vi "LabviewAMADTest.vi"() -> ()   [LabVIEW 2017]
uses:
  ADAM-4050DLL.dll
panel:
  in  "值_7":bool
  in  "DO7":bool
  in  "值_6":bool
  in  "DO6":bool
  in  "值_5":bool
  in  "DO5":bool
  in  "值_4":bool
  in  "DO4":bool
  in  "值_3":bool
  in  "DO3":bool
  in  "值_2":bool
  in  "DO2":bool
  in  "?":bool
  in  "DO1":bool
  out "inputresut":string[](array[string])
  in  "input":bool[](array[boolean])=[FALSE, FALSE, FALSE, FALSE, FALSE, FALSE, FALSE, FALSE]
  in  "?":bool
  in  "DO0":bool
  in  "停止 2":bool
  out "str_DO":string[](array[string])
  out "str_DI":string[](array[string])
  in  "停止":bool
  out "m_iDOTotalX":i32
  out "m_iDITotalX":i32
  # "值_0"
  # "值_1"
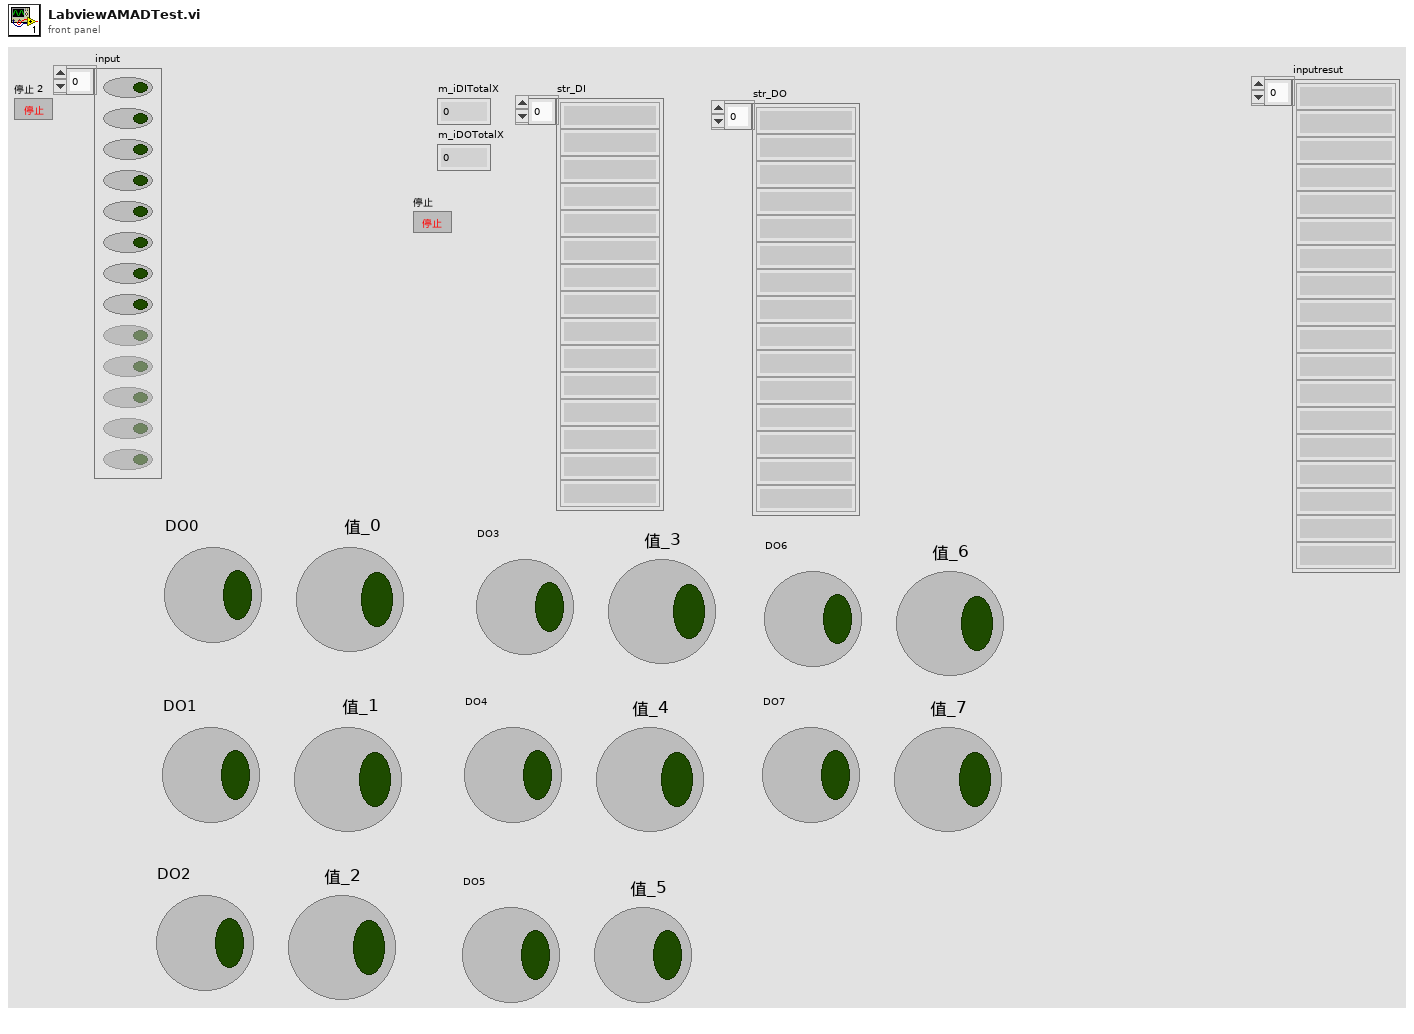
[diagram p1: front panel]
types:
  T1 = typedef "Semaphore RefNum" = refnum<k1>
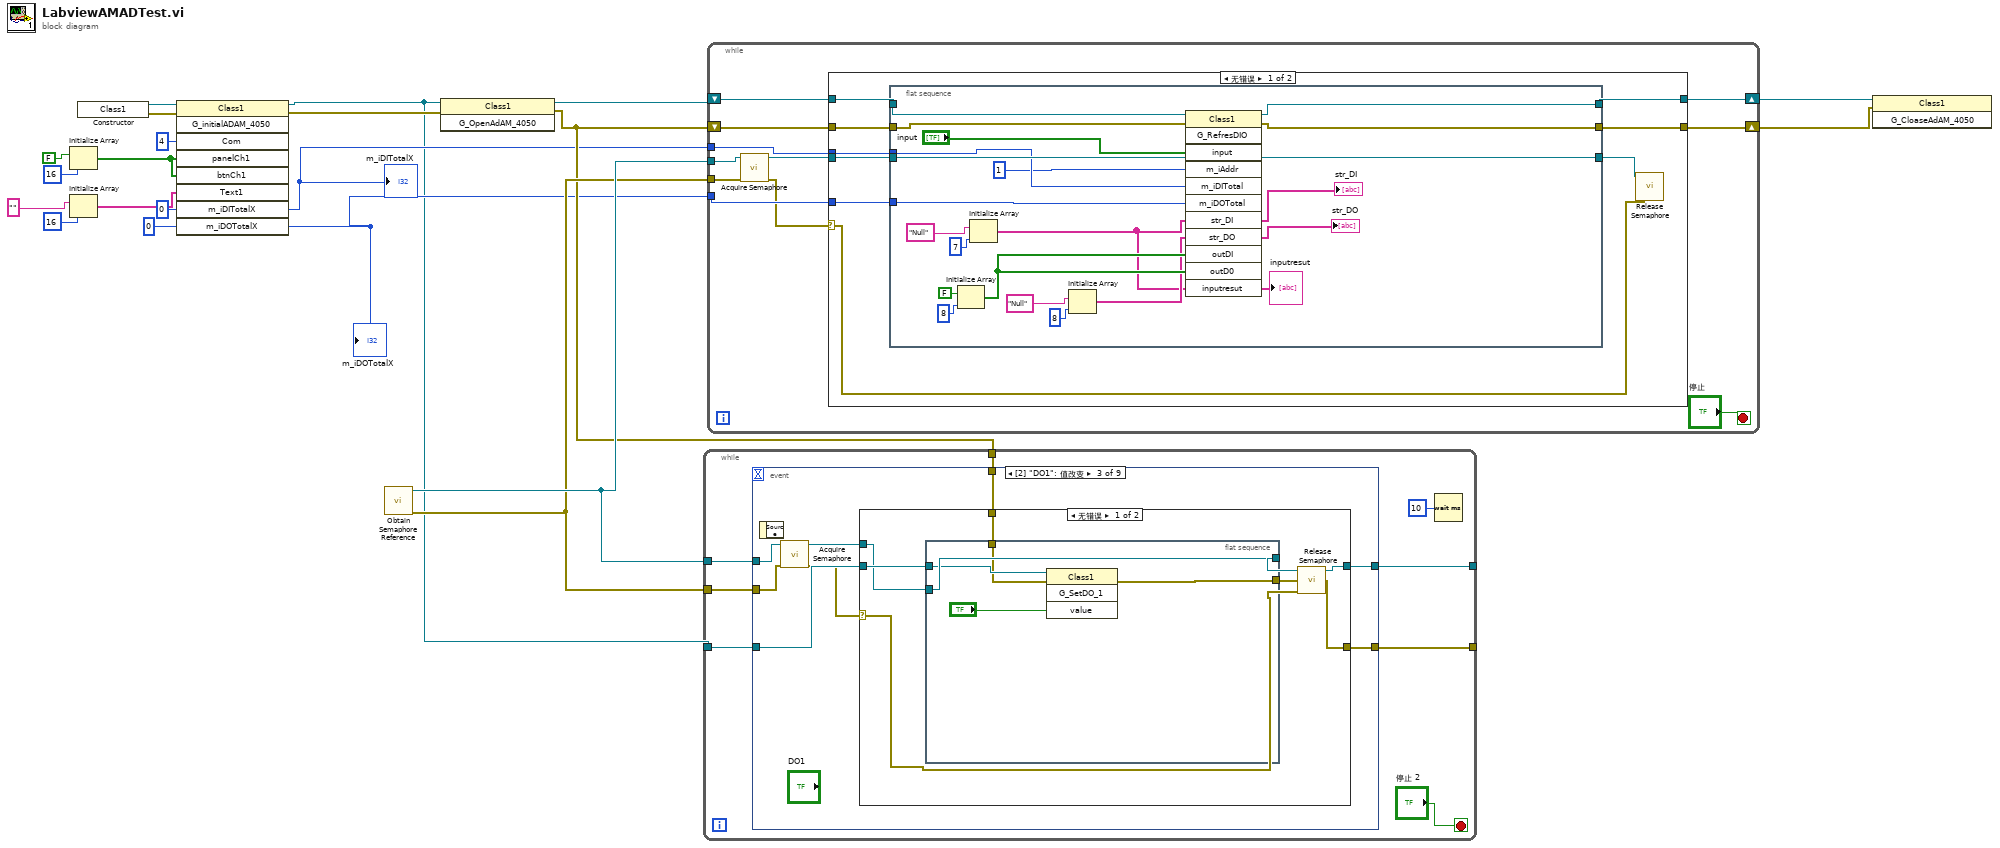
[diagram p0: block diagram]
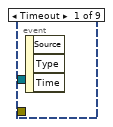
[diagram p2: hidden frame]
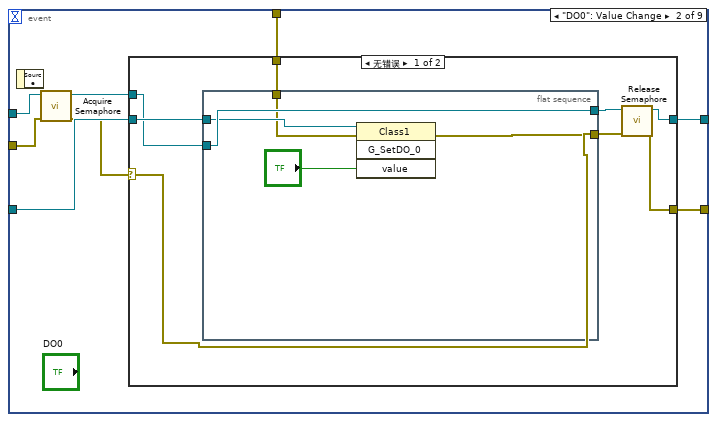
[diagram p3: hidden frame]
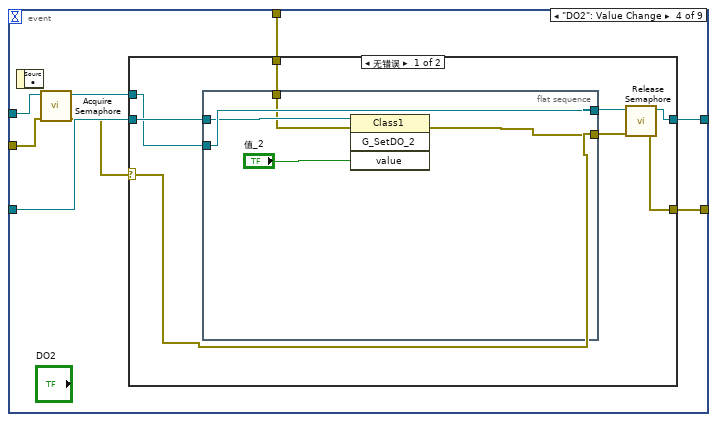
[diagram p6: hidden frame]
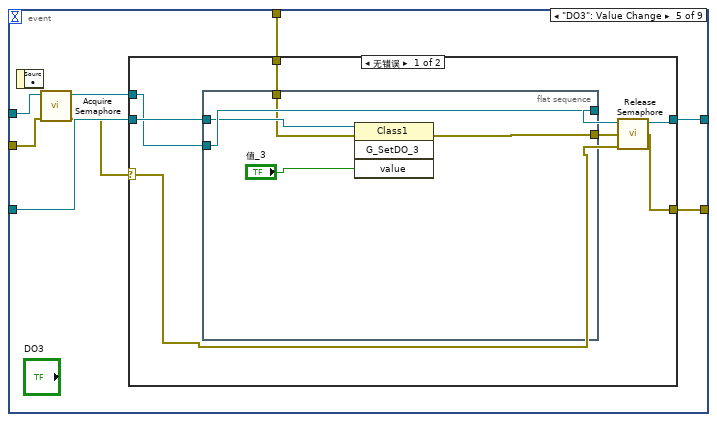
[diagram p8: hidden frame]
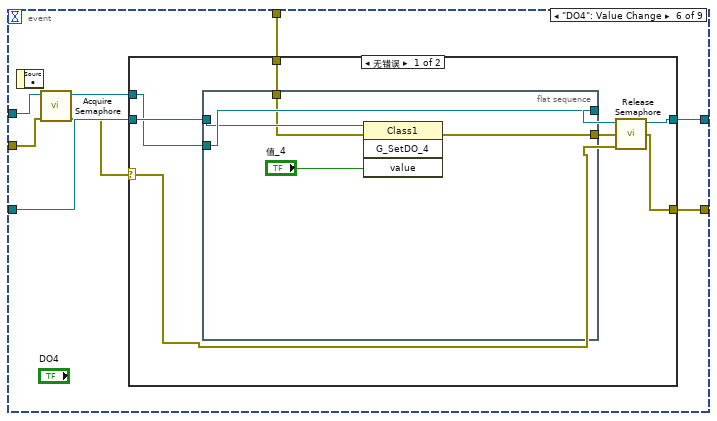
[diagram p10: hidden frame]
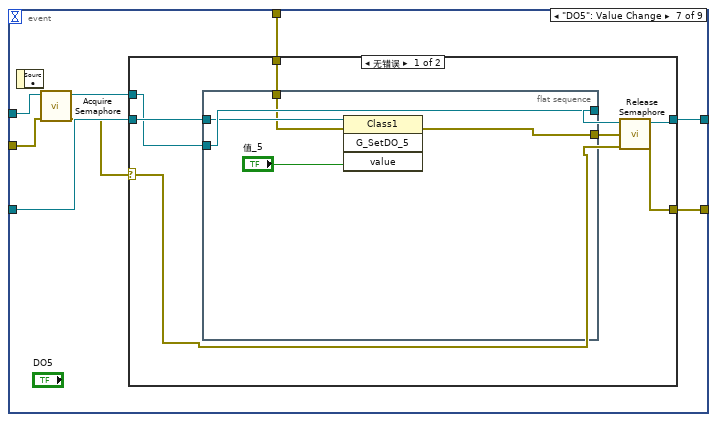
[diagram p12: hidden frame]
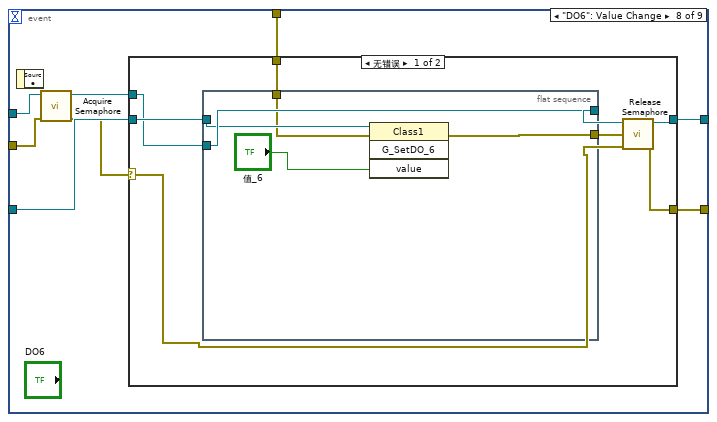
[diagram p14: hidden frame]
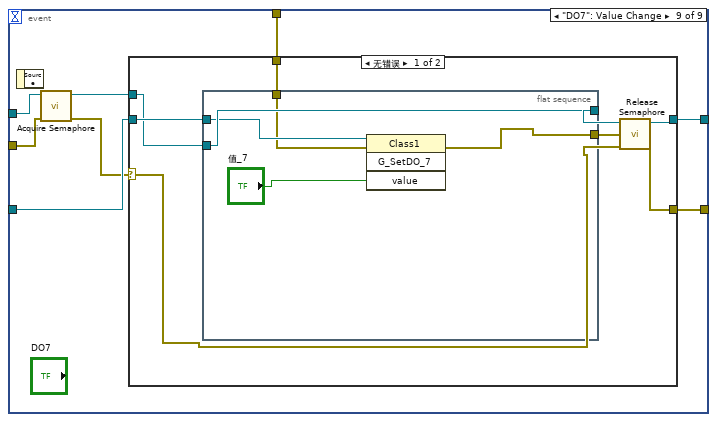
[diagram p16: hidden frame]
diagram:
  n1 = Initialize Array(FALSE, 16 ("维数大小")) -> (w16:bool[])
  n2 = Initialize Array("", 16 ("维数大小")) -> (w13:string[])
  n3 = constructor class="Class1"() -> (reference out=w21:refnum<k24>, error out=w20:errorcluster)  [unwired: 3 in, 1 out]
  n4 = invoke on="调用节点" class="Class1" method="G_initialADAM_4050"(reference=w21, error in=w20, "Com"=4, "panelCh1"=w16, "btnCh1"=w16, "Text1"=w13, "m_iDITotalX"=0, "m_iDOTotalX"=0) -> (reference out=w1:refnum<k24>, error out=w10:errorcluster, "m_iDITotalX"=w5:i32, "m_iDOTotalX"=w4:i32)  [unwired: 1 in, 5 out]
  "m_iDITotalX" <- w5
  "m_iDOTotalX" <- w4
  n5 = call <vilib>:"Obtain Semaphore Reference.vi"() -> ("error out"=w8:errorcluster, "semaphore"=w9:T1)  [unwired: 5 in, 1 out]
  n6 = invoke on="调用节点" class="Class1" method="G_OpenAdAM_4050"(reference=w1, error in=w10) -> (reference out=w7:refnum<k24>, error out=w6:errorcluster)  [unwired: 1 in, 1 out]
  n7 = while {
    tunnel: w9 -> [w27]
    tunnel: w8 -> [w26]
    tunnel: w1 -> [w25]
    tunnel: w6 -> [w24]
    tunnel: [w23] -> _
    tunnel: [w22] -> _
    stop <- "停止 2" stop-if-true
    n8 = event shown="[2] \"DO1\": 值改变" {
      selector: _ -> [_ _ _ _ _ _ _ _ _]
      dyn-events: _ -> [_ _ _ _ _ _ _ _ _]
      timeout: _ -> [_ _ _ _ _ _ _ _ _]
      tunnel: w27 -> [_ w36 w58 w80 w102 w124 w146 w168 w190]
      tunnel: w26 -> [_ w35 w57 w79 w101 w123 w145 w167 w189]
      tunnel: w25 -> [_ w37 w59 w81 w103 w125 w147 w169 w191]
      tunnel: w24 -> [_ w32 w54 w76 w98 w120 w142 w164 w186]
      tunnel: [_ w31 w53 w75 w97 w119 w141 w163 w185] -> w23
      tunnel: [_ w30 w52 w74 w96 w118 w140 w162 w184] -> w22
      event Timeout {
        n9 = event-data() -> ()  [unwired: 1 in, 3 out]
      }
      event "DO0": Value Change {
        n10 = event-data() -> ()  [unwired: 1 in, 1 out]
        n11 = call <vilib>:"Acquire Semaphore.vi"("error in (no error)"=w35, "semaphore"=w36) -> ("error out"=w33:errorcluster, "semaphore out"=w34:T1)  [unwired: 3 in, 1 out]
        n12 = case shown="无错误" w33 {
          selector: w33 -> [w43 w51]
          tunnel: w37 -> [w44 _]
          tunnel: w34 -> [w41 w50]
          tunnel: w32 -> [w40 _]
          tunnel: [w38 w50] -> w31
          tunnel: [w39 w51] -> w30
          frame No Error {
            n13 = flat-sequence {
              tunnel: w44 -> [w48]
              tunnel: w41 -> [w49]
              tunnel: [w49] -> w42
              tunnel: w40 -> [w47]
              tunnel: [w46] -> w39
              frame #0 {
                n14 = invoke class="Class1" method="G_SetDO_0"(reference=w48, error in=w47, "value"="?") -> (error out=w46:errorcluster)  [unwired: 1 in, 3 out]
              }
            }
            n15 = call <vilib>:"Release Semaphore.vi"("error in (no error)"=w43, "semaphore"=w42) -> ("semaphore out"=w38:T1)  [unwired: 4 in, 1 out]
          }
          frame Error {
          }
        }
      }
      event "DO1": Value Change {
        n16 = event-data() -> ()  [unwired: 1 in, 1 out]
        n17 = call <vilib>:"Acquire Semaphore.vi"("error in (no error)"=w57, "semaphore"=w58) -> ("error out"=w55:errorcluster, "semaphore out"=w56:T1)  [unwired: 3 in, 1 out]
        n18 = case shown="无错误" w55 {
          selector: w55 -> [w65 w73]
          tunnel: w59 -> [w66 _]
          tunnel: w56 -> [w63 w72]
          tunnel: w54 -> [w62 _]
          tunnel: [w60 w72] -> w53
          tunnel: [w61 w73] -> w52
          frame No Error {
            n19 = flat-sequence {
              tunnel: w66 -> [w70]
              tunnel: w63 -> [w71]
              tunnel: [w71] -> w64
              tunnel: w62 -> [w69]
              tunnel: [w68] -> w61
              frame #0 {
                n20 = invoke class="Class1" method="G_SetDO_1"(reference=w70, error in=w69, "value"="?") -> (error out=w68:errorcluster)  [unwired: 1 in, 3 out]
              }
            }
            n21 = call <vilib>:"Release Semaphore.vi"("error in (no error)"=w65, "semaphore"=w64) -> ("semaphore out"=w60:T1)  [unwired: 4 in, 1 out]
          }
          frame Error {
          }
        }
      }
      event "DO2": Value Change {
        n22 = event-data() -> ()  [unwired: 1 in, 1 out]
        n23 = call <vilib>:"Acquire Semaphore.vi"("error in (no error)"=w79, "semaphore"=w80) -> ("error out"=w77:errorcluster, "semaphore out"=w78:T1)  [unwired: 3 in, 1 out]
        n24 = case shown="无错误" w77 {
          selector: w77 -> [w87 w95]
          tunnel: w81 -> [w88 _]
          tunnel: w78 -> [w85 w94]
          tunnel: w76 -> [w84 _]
          tunnel: [w82 w94] -> w75
          tunnel: [w83 w95] -> w74
          frame No Error {
            n25 = flat-sequence {
              tunnel: w88 -> [w92]
              tunnel: w85 -> [w93]
              tunnel: [w93] -> w86
              tunnel: w84 -> [w91]
              tunnel: [w90] -> w83
              frame #0 {
                n26 = invoke class="Class1" method="G_SetDO_2"(reference=w92, error in=w91, "value"="值_2") -> (error out=w90:errorcluster)  [unwired: 1 in, 3 out]
              }
            }
            n27 = call <vilib>:"Release Semaphore.vi"("error in (no error)"=w87, "semaphore"=w86) -> ("semaphore out"=w82:T1)  [unwired: 4 in, 1 out]
          }
          frame Error {
          }
        }
      }
      event "DO3": Value Change {
        n28 = event-data() -> ()  [unwired: 1 in, 1 out]
        n29 = call <vilib>:"Acquire Semaphore.vi"("error in (no error)"=w101, "semaphore"=w102) -> ("error out"=w99:errorcluster, "semaphore out"=w100:T1)  [unwired: 3 in, 1 out]
        n30 = case shown="无错误" w99 {
          selector: w99 -> [w109 w117]
          tunnel: w103 -> [w110 _]
          tunnel: w100 -> [w107 w116]
          tunnel: w98 -> [w106 _]
          tunnel: [w104 w116] -> w97
          tunnel: [w105 w117] -> w96
          frame No Error {
            n31 = flat-sequence {
              tunnel: w110 -> [w114]
              tunnel: w107 -> [w115]
              tunnel: [w115] -> w108
              tunnel: w106 -> [w113]
              tunnel: [w112] -> w105
              frame #0 {
                n32 = invoke class="Class1" method="G_SetDO_3"(reference=w114, error in=w113, "value"="值_3") -> (error out=w112:errorcluster)  [unwired: 1 in, 3 out]
              }
            }
            n33 = call <vilib>:"Release Semaphore.vi"("error in (no error)"=w109, "semaphore"=w108) -> ("semaphore out"=w104:T1)  [unwired: 4 in, 1 out]
          }
          frame Error {
          }
        }
      }
      event "DO4": Value Change {
        n34 = event-data() -> ()  [unwired: 1 in, 1 out]
        n35 = call <vilib>:"Acquire Semaphore.vi"("error in (no error)"=w123, "semaphore"=w124) -> ("error out"=w121:errorcluster, "semaphore out"=w122:T1)  [unwired: 3 in, 1 out]
        n36 = case shown="无错误" w121 {
          selector: w121 -> [w131 w139]
          tunnel: w125 -> [w132 _]
          tunnel: w122 -> [w129 w138]
          tunnel: w120 -> [w128 _]
          tunnel: [w126 w138] -> w119
          tunnel: [w127 w139] -> w118
          frame No Error {
            n37 = flat-sequence {
              tunnel: w132 -> [w136]
              tunnel: w129 -> [w137]
              tunnel: [w137] -> w130
              tunnel: w128 -> [w135]
              tunnel: [w134] -> w127
              frame #0 {
                n38 = invoke class="Class1" method="G_SetDO_4"(reference=w136, error in=w135, "value"="值_4") -> (error out=w134:errorcluster)  [unwired: 1 in, 3 out]
              }
            }
            n39 = call <vilib>:"Release Semaphore.vi"("error in (no error)"=w131, "semaphore"=w130) -> ("semaphore out"=w126:T1)  [unwired: 4 in, 1 out]
          }
          frame Error {
          }
        }
      }
      event "DO5": Value Change {
        n40 = event-data() -> ()  [unwired: 1 in, 1 out]
        n41 = call <vilib>:"Acquire Semaphore.vi"("error in (no error)"=w145, "semaphore"=w146) -> ("error out"=w143:errorcluster, "semaphore out"=w144:T1)  [unwired: 3 in, 1 out]
        n42 = case shown="无错误" w143 {
          selector: w143 -> [w153 w161]
          tunnel: w147 -> [w154 _]
          tunnel: w144 -> [w151 w160]
          tunnel: w142 -> [w150 _]
          tunnel: [w148 w160] -> w141
          tunnel: [w149 w161] -> w140
          frame No Error {
            n43 = flat-sequence {
              tunnel: w154 -> [w158]
              tunnel: w151 -> [w159]
              tunnel: [w159] -> w152
              tunnel: w150 -> [w157]
              tunnel: [w156] -> w149
              frame #0 {
                n44 = invoke class="Class1" method="G_SetDO_5"(reference=w158, error in=w157, "value"="值_5") -> (error out=w156:errorcluster)  [unwired: 1 in, 3 out]
              }
            }
            n45 = call <vilib>:"Release Semaphore.vi"("error in (no error)"=w153, "semaphore"=w152) -> ("semaphore out"=w148:T1)  [unwired: 4 in, 1 out]
          }
          frame Error {
          }
        }
      }
      event "DO6": Value Change {
        n46 = event-data() -> ()  [unwired: 1 in, 1 out]
        n47 = call <vilib>:"Acquire Semaphore.vi"("error in (no error)"=w167, "semaphore"=w168) -> ("error out"=w165:errorcluster, "semaphore out"=w166:T1)  [unwired: 3 in, 1 out]
        n48 = case shown="无错误" w165 {
          selector: w165 -> [w175 w183]
          tunnel: w169 -> [w176 _]
          tunnel: w166 -> [w173 w182]
          tunnel: w164 -> [w172 _]
          tunnel: [w170 w182] -> w163
          tunnel: [w171 w183] -> w162
          frame No Error {
            n49 = flat-sequence {
              tunnel: w176 -> [w180]
              tunnel: w173 -> [w181]
              tunnel: [w181] -> w174
              tunnel: w172 -> [w179]
              tunnel: [w178] -> w171
              frame #0 {
                n50 = invoke class="Class1" method="G_SetDO_6"(reference=w180, error in=w179, "value"="值_6") -> (error out=w178:errorcluster)  [unwired: 1 in, 3 out]
              }
            }
            n51 = call <vilib>:"Release Semaphore.vi"("error in (no error)"=w175, "semaphore"=w174) -> ("semaphore out"=w170:T1)  [unwired: 4 in, 1 out]
          }
          frame Error {
          }
        }
      }
      event "DO7": Value Change {
        n52 = event-data() -> ()  [unwired: 1 in, 1 out]
        n53 = call <vilib>:"Acquire Semaphore.vi"("error in (no error)"=w189, "semaphore"=w190) -> ("error out"=w187:errorcluster, "semaphore out"=w188:T1)  [unwired: 3 in, 1 out]
        n54 = case shown="无错误" w187 {
          selector: w187 -> [w197 w205]
          tunnel: w191 -> [w198 _]
          tunnel: w188 -> [w195 w204]
          tunnel: w186 -> [w194 _]
          tunnel: [w192 w204] -> w185
          tunnel: [w193 w205] -> w184
          frame No Error {
            n55 = flat-sequence {
              tunnel: w198 -> [w202]
              tunnel: w195 -> [w203]
              tunnel: [w203] -> w196
              tunnel: w194 -> [w201]
              tunnel: [w200] -> w193
              frame #0 {
                n56 = invoke class="Class1" method="G_SetDO_7"(reference=w202, error in=w201, "value"="值_7") -> (error out=w200:errorcluster)  [unwired: 1 in, 3 out]
              }
            }
            n57 = call <vilib>:"Release Semaphore.vi"("error in (no error)"=w197, "semaphore"=w196) -> ("semaphore out"=w192:T1)  [unwired: 4 in, 1 out]
          }
          frame Error {
          }
        }
      }
    }
    n58 = Wait (ms)(milliseconds to wait=u32 10 ("等待时间（毫秒）")) -> ()  [unwired: 1 out]
  }
  n59 = while {
    shift-right: [w214] -> w3
    shift-left: w7 -> [w216]
    shift-right: [w213] -> w2
    shift-left: w6 -> [w215]
    tunnel: w5 -> [w211]
    tunnel: w4 -> [w210]
    tunnel: w9 -> [w208]
    tunnel: w8 -> [w207]
    stop <- "停止" stop-if-true
    n60 = call <vilib>:"Acquire Semaphore.vi"("error in (no error)"=w207, "semaphore"=w208) -> ("error out"=w209:errorcluster, "semaphore out"=w206:T1)  [unwired: 3 in, 1 out]
    n61 = case shown="无错误" w209 {
      selector: w209 -> [w217 _]
      tunnel: w216 -> [w225 w248]
      tunnel: w215 -> [w224 w247]
      tunnel: [w223 w248] -> w214
      tunnel: [w222 w247] -> w213
      tunnel: w211 -> [w221 _]
      tunnel: w210 -> [w220 _]
      tunnel: w206 -> [w219 _]
      frame No Error {
        n62 = flat-sequence {
          tunnel: w225 -> [w246]
          tunnel: w224 -> [w245]
          tunnel: [w233] -> w223
          tunnel: [w244] -> w222
          tunnel: w221 -> [w237]
          tunnel: w220 -> [w236]
          tunnel: [w239] -> w218
          tunnel: w219 -> [w239]
          frame #0 {
            n63 = Initialize Array(FALSE, 8 ("维数大小")) -> (w238:bool[])
            n64 = Initialize Array("Null", 7 ("维数大小")) -> (w228:string[])
            n65 = Initialize Array("Null", 8 ("维数大小")) -> (w229:string[])
            n66 = invoke class="Class1" method="G_RefresDIO"(reference=w246, error in=w245, "input"="input", "m_iAddr"=1, "m_iDITotal"=w237, "m_iDOTotal"=w236, "str_DI"=w228, "str_DO"=w229, "outDI"=w238, "outD0"=w238, "inputresut"=w228) -> (reference out=w233:refnum<k24>, error out=w244:errorcluster, "str_DI"=→"str_DI":string[], "str_DO"=→"str_DO":string[], "inputresut"=→"inputresut":string[])  [unwired: 1 in, 7 out]
          }
        }
        n67 = call <vilib>:"Release Semaphore.vi"("error in (no error)"=w217, "semaphore"=w218) -> ()  [unwired: 4 in, 2 out]
      }
      frame Error {
      }
    }
  }
  n68 = invoke on="调用节点" class="Class1" method="G_CloaseAdAM_4050"(reference=w3, error in=w2) -> ()  [unwired: 1 in, 3 out]
